vi "tpg361_get_p.vi"(5 "tpg361_delay 3":u32=500, 6 "err_in":errorcluster, 7 "tpg361_delay":u32=500, 8 "tpg361_delay 2":u32=500, 10 "tpg361_visa":refnum<visa-resource-name>) -> (0 "err_out":errorcluster, 3 "Pressure (Torr)":string)   [LabVIEW 2019]
panel:
  out "Overall Status":bool
  out "Acknowledgement Status":bool
  out "tpg361_visa 2":refnum<visa-resource-name>
  in  "tpg361_b2r 2":u32
  in  "tpg361_b2r":u32
  # "VISA"
  # "DELAY"
  # "BYTE AT PORT"
  # "STATUS"
  # "ERROR"
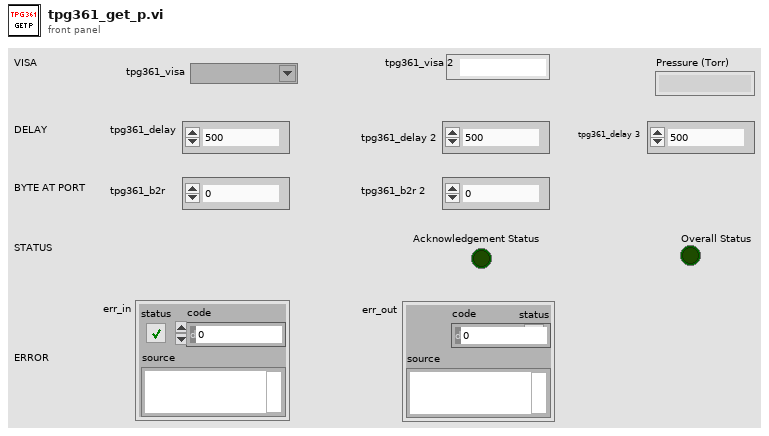
[diagram p1: front panel]
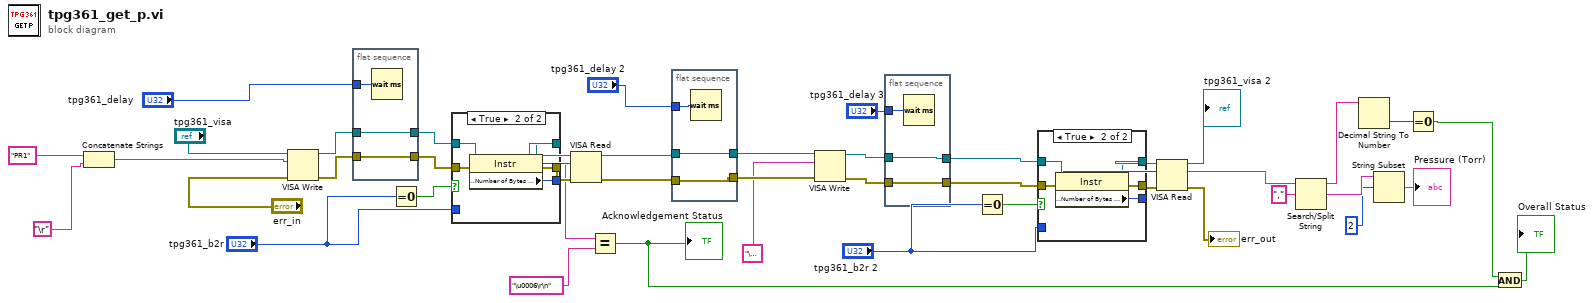
[diagram p0: block diagram]
diagram:
  n1 = Concatenate Strings("PR1" ("string"), "\r") -> (w17:string)
  n2 = VISA Write(VISA resource name="tpg361_visa", write buffer=w17, error in (no error)="err_in") -> (VISA resource name out=w43:refnum<visa-resource-name>, error out=w45:errorcluster)  [unwired: 1 out]
  n3 = flat-sequence {
    tunnel: w45 -> [w47]
    tunnel: [w47] -> w44
    tunnel: w43 -> [w46]
    tunnel: [w46] -> w42
    tunnel: "tpg361_delay" -> [w48]
    frame #0 {
      n4 = Wait (ms)(milliseconds to wait=w48) -> ()  [unwired: 1 out]
    }
  }
  n5 = Equal To 0?(x="tpg361_b2r") -> (x = 0?=w38:bool)
  n6 = case shown="True" w38 {
    tunnel: w44 -> [w50 w56]
    tunnel: w42 -> [w51 w55]
    tunnel: [w51 w54] -> w36
    tunnel: [w50 w53] -> w35
    tunnel: [w49 w52] -> w34
    tunnel: "tpg361_b2r" -> [w49 _]
    frame False {
    }
    frame True {
      n7 = property class="Instr"(reference=w55, error in=w56) -> (reference out=w54:refnum<visa-resource-name>, error out=w53:errorcluster, "Serial Settings:Number of Bytes at Serial Port"=w52:u32)
    }
  }
  n8 = VISA Read(VISA resource name=w36, byte count=w34, error in (no error)=w35) -> (VISA resource name out=w33:refnum<visa-resource-name>, read buffer=w7:string, error out=w32:errorcluster)  [unwired: 1 out]
  n9 = Equal?(x=w7, y="\u0006\r\n") -> (x = y?=w2:bool)
  "Acknowledgement Status" <- w2
  n10 = flat-sequence {
    tunnel: [w57] -> w30
    tunnel: w33 -> [w59]
    tunnel: [w59] -> w31
    tunnel: "tpg361_delay 2" -> [w58]
    tunnel: w32 -> [w57]
    frame #0 {
      n11 = Wait (ms)(milliseconds to wait=w58) -> ()  [unwired: 1 out]
    }
  }
  n12 = VISA Write(VISA resource name=w31, write buffer="\u0005", error in (no error)=w30) -> (VISA resource name out=w23:refnum<visa-resource-name>, error out=w22:errorcluster)  [unwired: 1 out]
  n13 = flat-sequence {
    tunnel: [w61] -> w29
    tunnel: [w62] -> w28
    tunnel: w23 -> [w62]
    tunnel: w22 -> [w61]
    tunnel: "tpg361_delay 3" -> [w60]
    frame #0 {
      n14 = Wait (ms)(milliseconds to wait=w60) -> ()  [unwired: 1 out]
    }
  }
  n15 = Equal To 0?(x="tpg361_b2r 2") -> (x = 0?=w27:bool)
  n16 = case shown="True" w27 {
    tunnel: w29 -> [w64 w70]
    tunnel: w28 -> [w65 w69]
    tunnel: [w65 w68] -> w26
    tunnel: [w64 w67] -> w25
    tunnel: [w63 w66] -> w24
    tunnel: "tpg361_b2r 2" -> [w63 _]
    frame False {
    }
    frame True {
      n17 = property class="Instr"(reference=w69, error in=w70) -> (reference out=w68:refnum<visa-resource-name>, error out=w67:errorcluster, "Serial Settings:Number of Bytes at Serial Port"=w66:u32)
    }
  }
  n18 = VISA Read(VISA resource name=w26, byte count=w24, error in (no error)=w25) -> (VISA resource name out=→"tpg361_visa 2":refnum<visa-resource-name>, read buffer=w15:string, error out=→"err_out":errorcluster)  [unwired: 1 out]
  n19 = Search/Split String(string=w15, search string/char (-)=",") -> (substring before match=w10:string, match + rest of string=w13:string)  [unwired: 1 in, 1 out]
  n20 = Decimal String To Number(string=w10) -> (number=w9:i32)  [unwired: 2 in, 1 out]
  n21 = String Subset(string=w13, offset (0)=2) -> (substring=→"Pressure (Torr)":string)  [unwired: 1 in]
  n22 = Equal To 0?(x=w9) -> (x = 0?=w3:bool)
  n23 = And(x=w3, y=w2) -> (x .and. y?=→"Overall Status":bool)
